vi "macro_Rotation2d_X_Y.vi"   [LabVIEW 2019, in "Trajectory_Library.lvlib"]
uses:
  Trajectory_Library.lvlib
  Util_CalcDist.vi
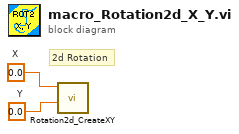
[diagram p0: block diagram]
diagram:
  w1 = 0.0  # X
  w2 = 0.0  # Y
  # "2d Rotation"
  n1 = call "Rotation2d_CreateXY.vi"("Y or sine"=w2, "X or  cosine"=w1) -> ()  [unwired: 9 in, 1 out]
